vi "LifetimePickTACCube.vi"(2 "notes 2":refnum<vi>, 3 "already x spots":i16) -> (1 "spots":i16)   [LabVIEW 2009]
uses:
  spotproperties.ctl
  <vilib>/vision/NI_Vision_Development_Module.lvlib
panel:
  out "TAC Intensity":u32[](array[numeric])
  out "Lifetime[ns]":ext[](array[numeric]) format="%.2f"
  out "tauerror":dbl[](array[numeric]) format="%.2f"
  out "last coordinates":i32[](array[numeric])
  out "F2-Value overall":dbl format="%.2f"
  out "nachträgliches markieren":i32[](array[numeric]) caption="Coordinates"
  in  "notes":string
  in  "spotsize":bool
  in  "spotsize (Pixel)":u16=10
  out "Intensity":u32[](array[numeric])
  in  "always store button":bool
  out "ALWAYS STORE?":bool
  in  "store this":bool
  out "always store":bool
  in  "Autoscale y":bool caption="Autoscale 2"
  in  "Autoscale":bool
  in  "plot":u16(ring) items=["linear y-axis", "log y-axis"]
  out "takeall?":bool
  out "F2-Value TAC":dbl caption="F2-Value" format="%.2f"
  in  "RGB/false color?":bool
  out "Decays":u32[][](graph)
  out "Tool":i32(ring) items=["Point", "Line", "Rectangle", "Oval", "Polygon", "Free", "Annulus", "Rotated Rectangle", "Zoom", "Pan", "MultiLine", "FreeLine"]
  out "Coordinates":i32[](array[numeric])
  out "Event":i32(ring) items=["No  event", "Click event", "Draw event", "Move event", "Size event", "Scroll event", "Activate event", "Close event", "Double click event"]
  in  "TAC Cube":T1(ring)
  in  "plane":u32
  in  "threshold":cluster{"max":u32, "min":u32} caption="Threshold"
  in  "stop":bool
  # "S"
  # "S"
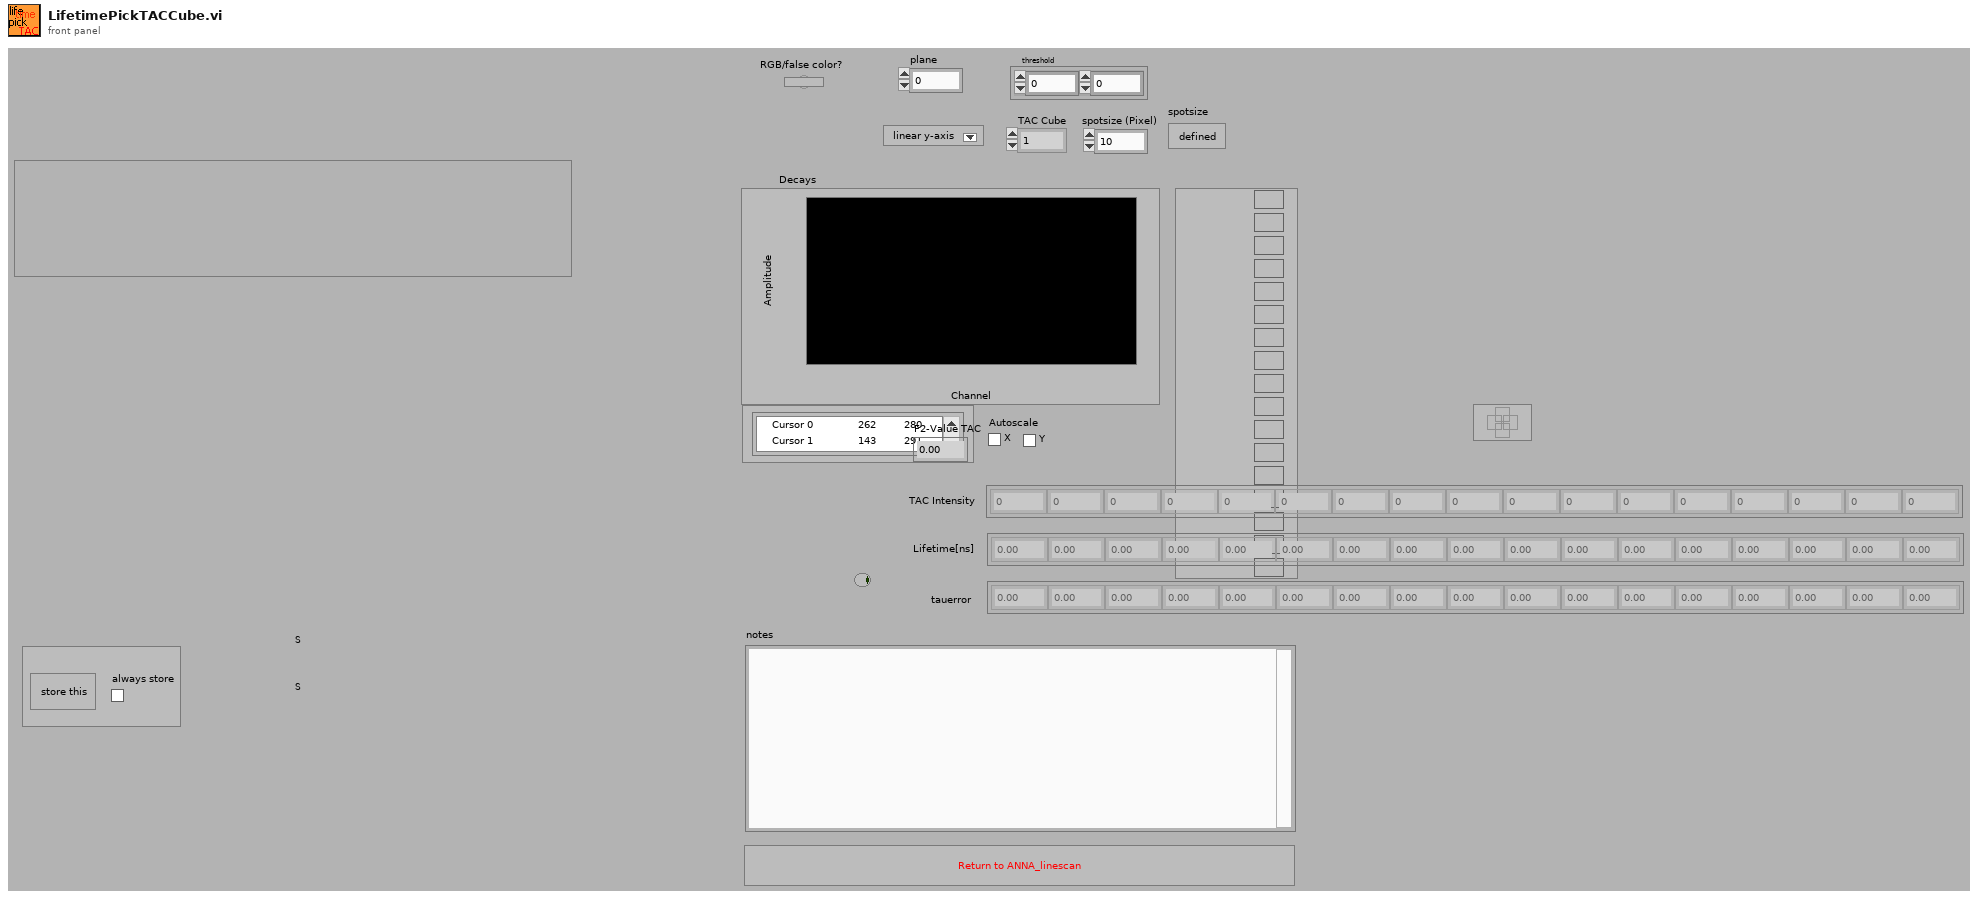
[diagram p1: front panel]
types:
  T1 = enum16{"1", "2", "3", "4", "5", "6", "7", "Sum", "Sep."}
  T2 = typedef "spotproperties.ctl" = cluster{"draw?":bool, "plane":u32, "Coordinates":i32[], "TACWindow":cluster{"TACWindow1":i32, "TACWindow2":i32}, "Lifetime[ns]":ext[], "tauerror":dbl[], "F2-Value overall":dbl, "overall intensity":u32[], "F2-Value TAC":dbl, "TAC intensity":u32[], "Decay":u32[][]}
  T3 = enum16{"Ini", "Get", "Set", "Refresh", "dump", "move", "name"}
  T4 = typedef "FIFOSettings_BH.ctt" = cluster{"Measurement":cluster{"Binning (ms)":sgl, "External Trigger Condition":u16, "Stop Condition:":u16, "Stop Count":dbl, "Buffer Size (Photons)":u16, "No of Channels":u16, "Ext Latch Delay":i16}, "ADC":cluster{"Module":u16, "ADC Resolution":i32, "Dither Range":i16, "Count Increment":i16, "Macro Time Clock":i16}, "SYNC":cluster{"SYNC ZC Level (mV)":sgl, "SYNC Freq Divider":i16, "SYNC Holdoff (ns)":sgl, "SYNC Threshold (mV)":sgl}, "TAC":cluster{"TAC Range (ns)":sgl, "TAC Gain":i16, "TAC Offset (%)":sgl, "TAC Limit Low (%)":sgl, "TAC Limit High (%)":sgl}, "CFD":cluster{"CFD Limit Low (mV)":sgl, "CFD Limit High (mV)":sgl, "CFD ZC Level (mV)":sgl, "CFD Holdoff (ns)":sgl}}
  T5 = typedef "Settings.ctl" = cluster{"threshold":cluster{"max":u32, "min":u32}, "RGB or false color":bool, "16bit":bool, "log/lin axis":u16, "spotsize button":bool, "Pixelsize":u16, "autoscale x":bool, "autoscale y":bool, "correlation":bool, "ADC-Resolution":i32, "F2-lifetime":cluster{"display tau":bool, "display F2":bool, "Palette Number lifetime":enum32{"Gray", "Binary", "Gradient", "Rainbow", "Temperature"}, "Palette Number F2":enum32{"Gray", "Binary", "Gradient", "Rainbow", "Temperature"}, "max tau-Value":dbl, "min tau-Value":dbl, "max F2-Value":dbl, "min F2-Value":dbl}, "TAC-Window 1":u16, "TAC-Window 2":u16, "false color palette":cluster{"1":u32, "2":u32, "3":u32, "4":u32, "5":u32, "6":u32, "7":u32, "8":u32, "8 2":u32, "8 3":u32, "8 4":u32, "8 5":u32}}
  T6 = enum32{"No Selection", "Point", "Line", "Rectangle", "Oval", "Polygon", "Free", "Unused1", "Zoom", "Unused2", "Broken Line", "Free Hand Line"}[]
  T7 = typedef "IMAQ Image.ctl" = refnum<image>
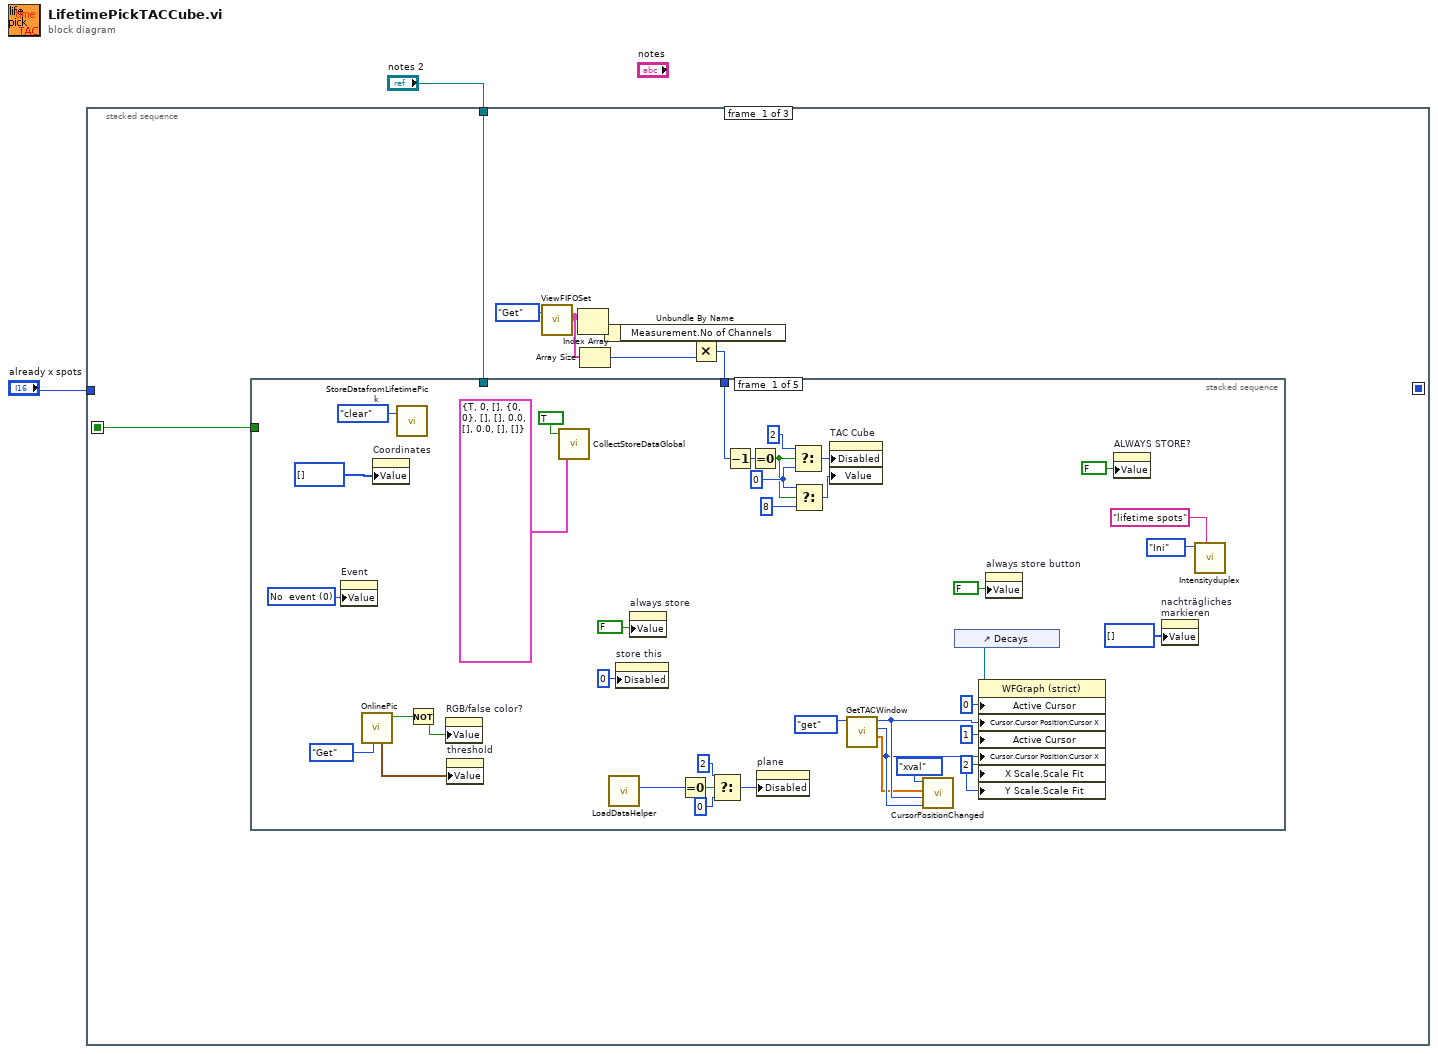
[diagram p0: block diagram]
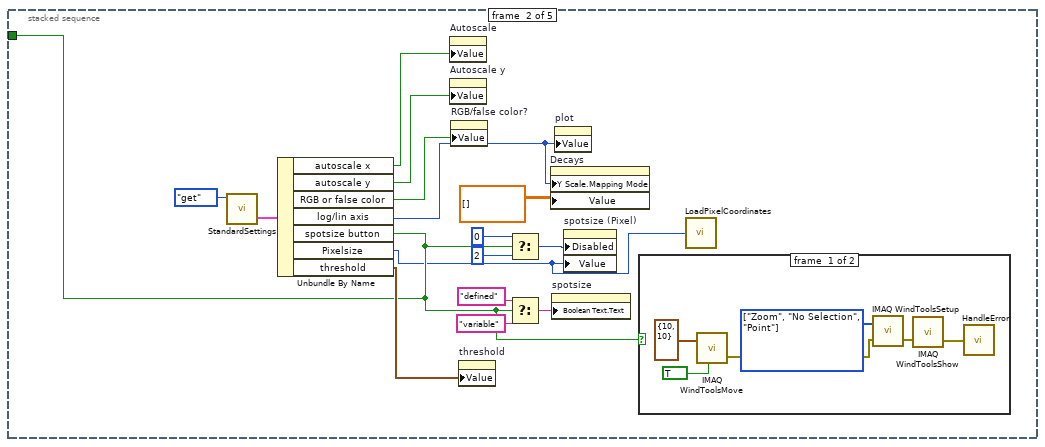
[diagram p2: hidden frame]
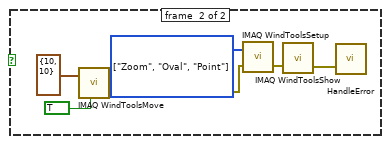
[diagram p3: hidden frame]
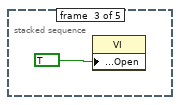
[diagram p4: hidden frame]
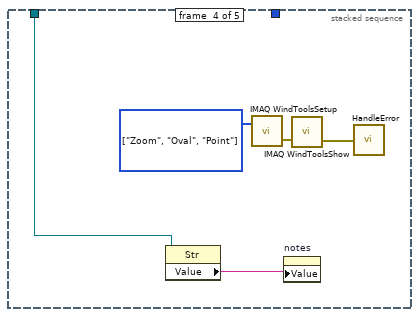
[diagram p5: hidden frame]
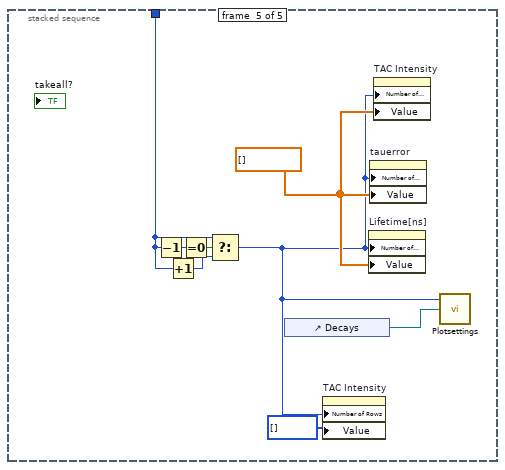
[diagram p6: hidden frame]
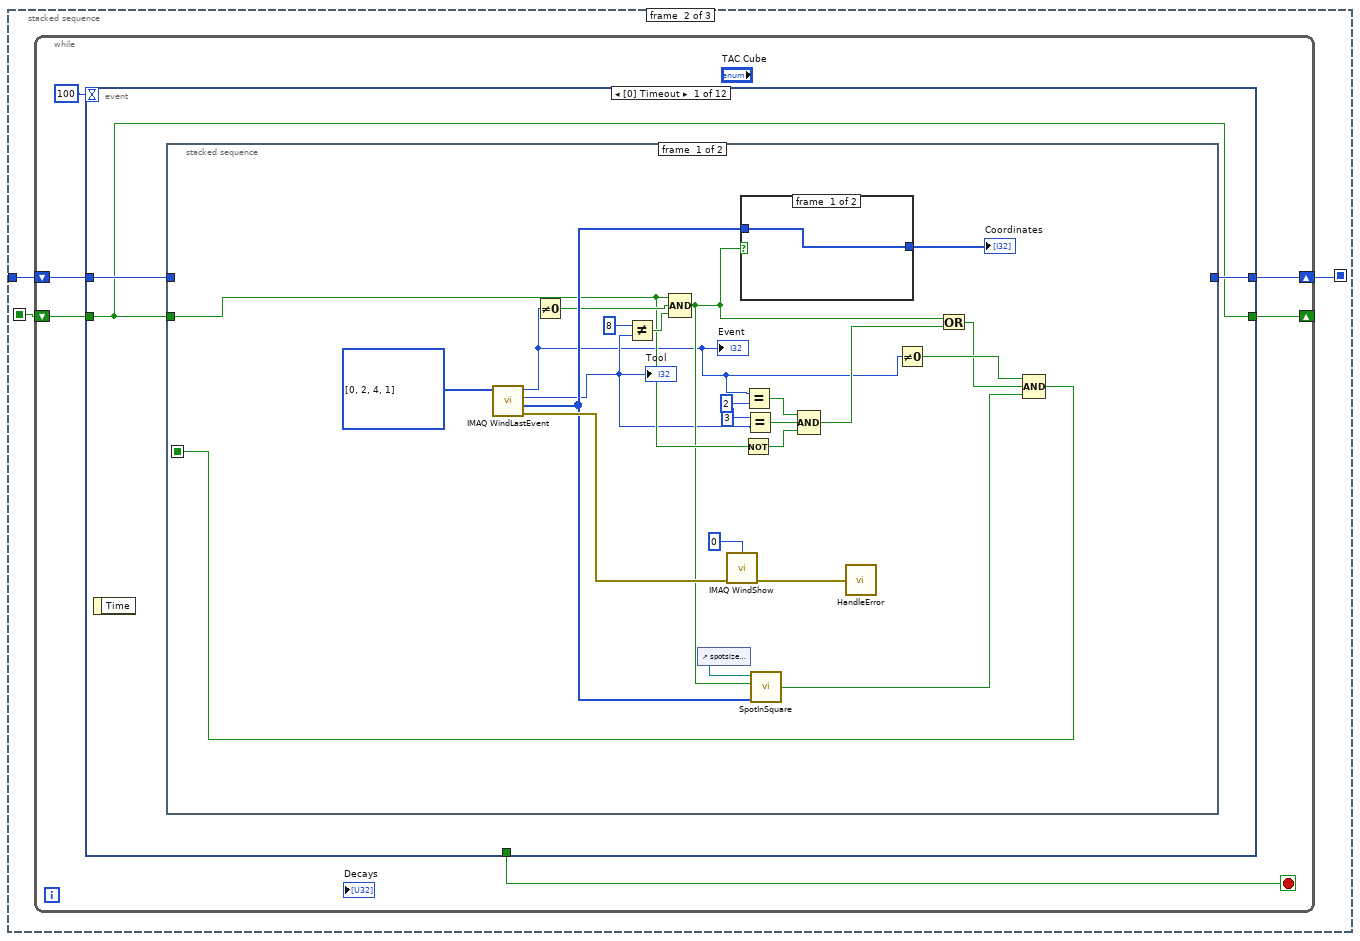
[diagram p7: hidden frame]
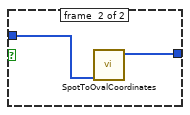
[diagram p8: hidden frame]
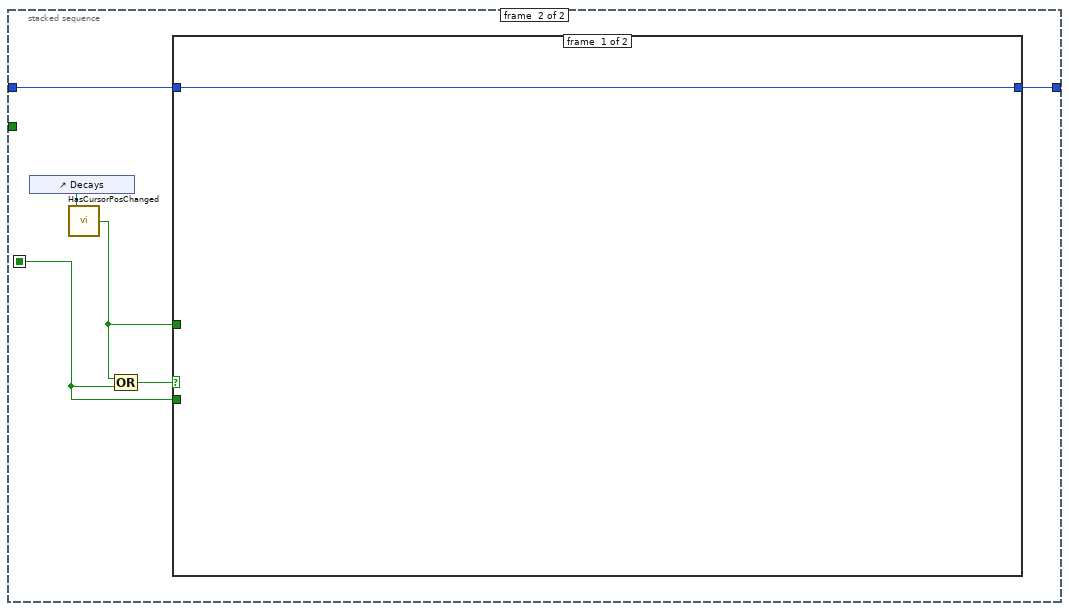
[diagram p9: hidden frame]
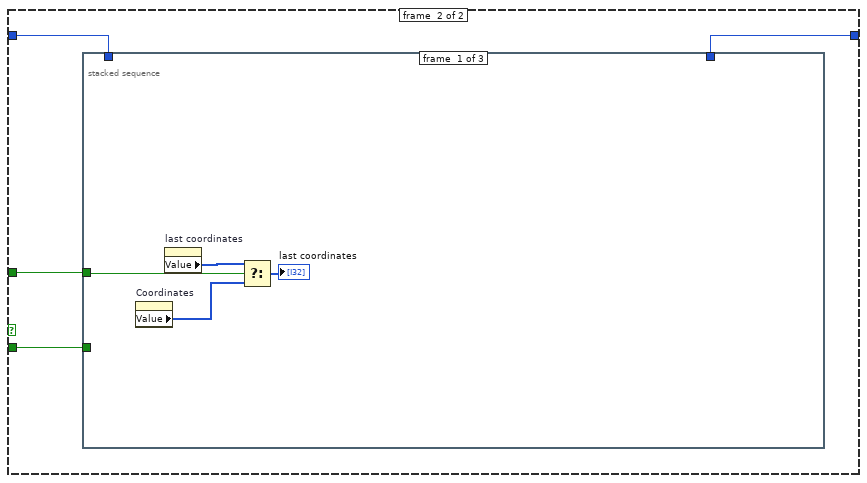
[diagram p10: hidden frame]
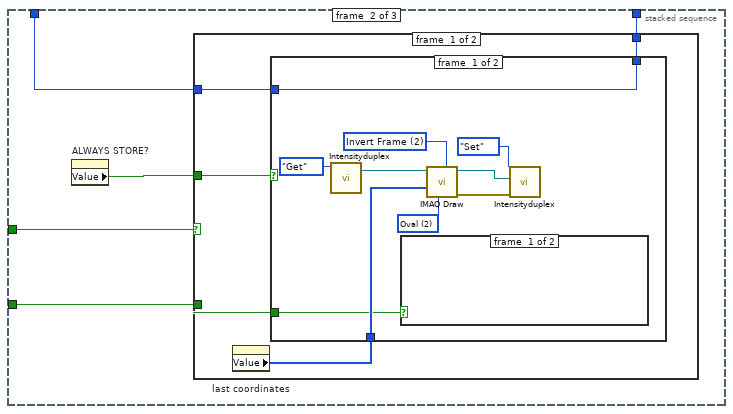
[diagram p11: hidden frame]
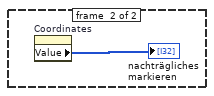
[diagram p12: hidden frame]
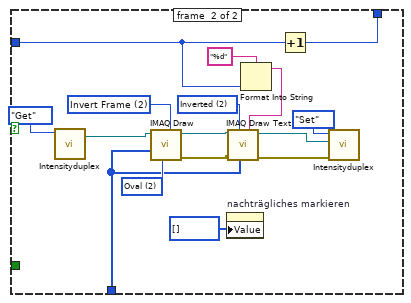
[diagram p13: hidden frame]
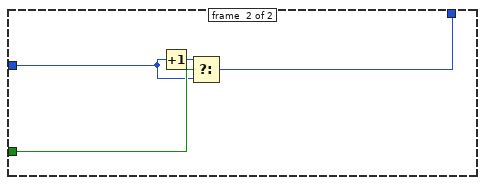
[diagram p14: hidden frame]
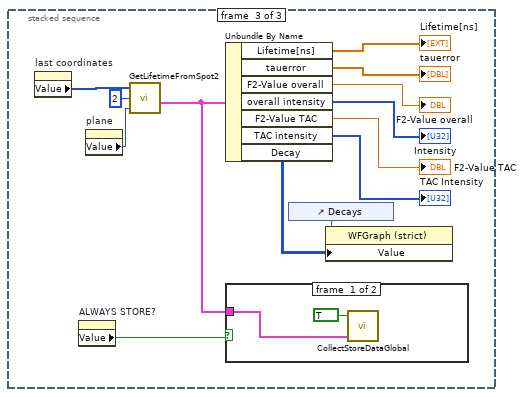
[diagram p15: hidden frame]
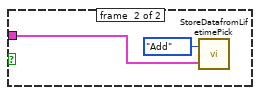
[diagram p16: hidden frame]
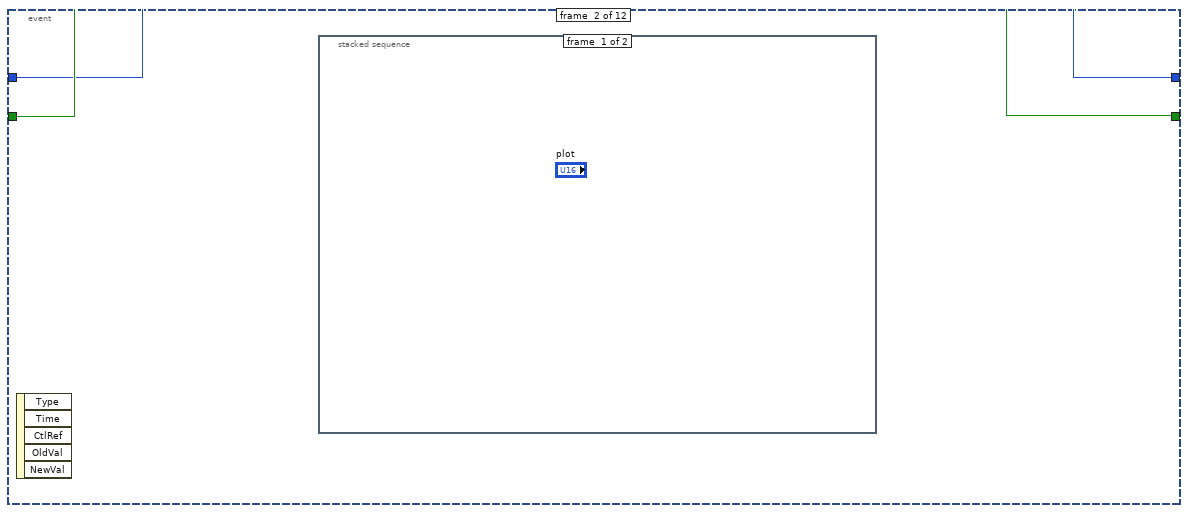
[diagram p17: hidden frame]
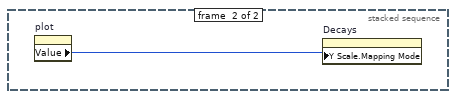
[diagram p18: hidden frame]
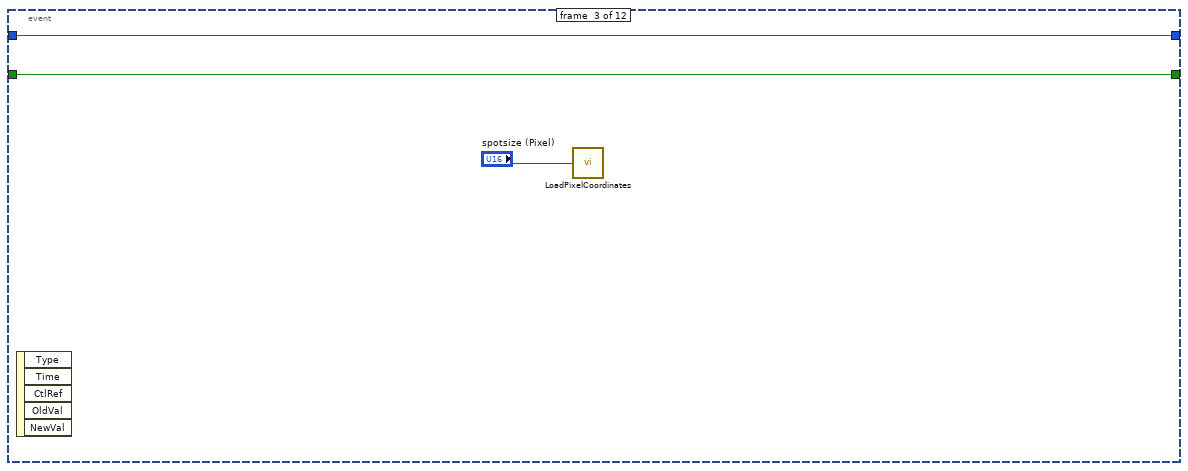
[diagram p19: hidden frame]
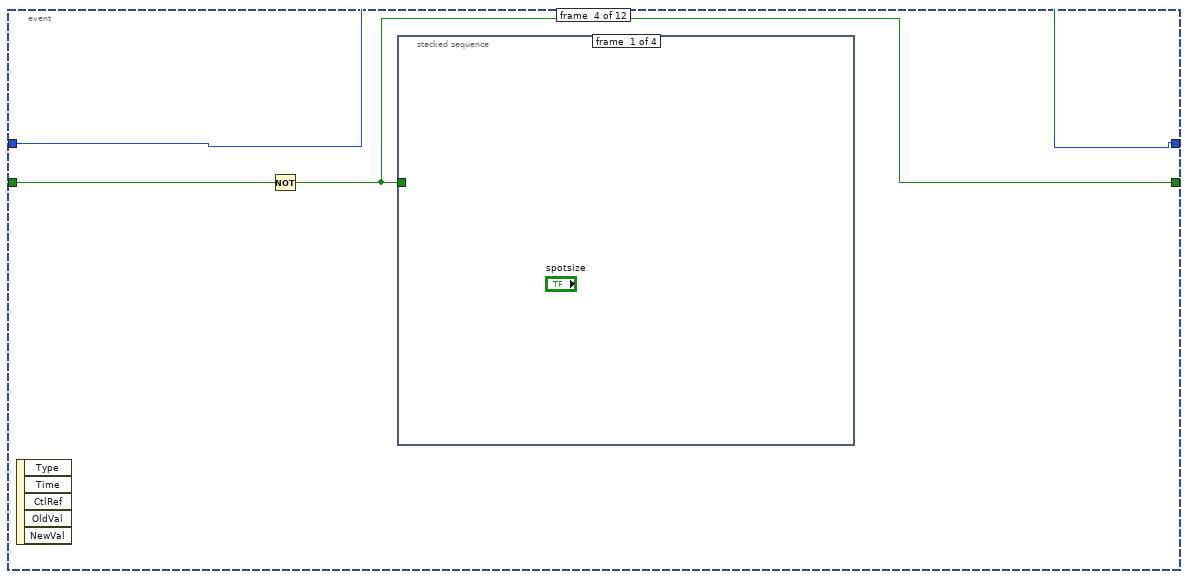
[diagram p20: hidden frame]
diagram:
  n1 = stacked-sequence {
    seq-local: [_ w92 _] -> [_ _ w345]
    seq-local: [w9 _ _] -> [_ w91 _]
    tunnel: "already x spots" -> [_ w93 _]
    tunnel: "notes 2" -> [w10 _ w347]
    frame #0 {
      n2 = call "ViewFIFOSet.vi"("Enum"=enum16{"Display", "change", "Get", "Set"}."Get") -> ("FIFO Settings (Array)"=w6:T4[])  [unwired: 1 in]
      n3 = Index Array(array=w6) -> (element=w7:T4)  [unwired: 1 in]
      n4 = Array Size(array=w6) -> (size(s)=w4:i32)
      n5 = Unbundle By Name(w7) -> ("Measurement.No of Channels"=w3:u16)
      n6 = Multiply(x=w3, y=w4) -> (x*y=w5:i32)
      n7 = stacked-sequence {
        tunnel: w10 -> [_ _ _ w79 _]
        tunnel: [_ w50 _ _ _] -> w9
        tunnel: w5 -> [w13 _ _ _ w86]
        frame #0 {
          w14 = u8 0 ("Disabled")
          w41 = 0 items=["No  event", "Click event", "Draw event", "Move event", "Size event", "Scroll event", "Activate event", "Close event", "Double click event"] ("Event")
          w45 = u8 2 ("X Scale.Scale Fit")
          n8 = property on="Event" class="Ring (strict)"("Value"=w41) -> ()  [unwired: 2 in, 2 out]
          n9 = call "OnlinePic.vi"("action"=enum16{"Get", "Set", "Change", "ini"}."Get" ("Enum")) -> ("RGB/False out"=w32:bool, "Threshold (max) OUT"=w33:cluster{"max":u32, "min":u32})  [unwired: 6 in, 3 out]
          n10 = property on="Coordinates" class="Array (strict)"("Value"=i32[] []) -> ()  [unwired: 2 in, 2 out]
          n11 = call "StoreDatafromLifetimePick.vi"("Enum"=enum16{"clear", "Get", "Set"}."clear") -> ()  [unwired: 1 in, 2 out]
          n12 = Not(x=w32) -> (.not. x?=w31:bool)
          n13 = property on="RGB/false color?" class="Bool (strict)"("Value"=w31) -> ()  [unwired: 2 in, 2 out]
          n14 = property on="threshold" class="Clust (strict)"("Value"=w33) -> ()  [unwired: 2 in, 2 out]
          n15 = call "CollectStoreDataGlobal.vi"("SpotProperties 2"=T2 {"draw?"=TRUE, "plane"=0, "Coordinates"=[], "TACWindow"={"TACWindow1"=0, "TACWindow2"=0}, "Lifetime[ns]"=[], "tauerror"=[], "F2-Value overall"=0.0, "overall intensity"=[], "F2-Value TAC"=0.0, "TAC intensity"=[], "Decay"=[]}, "set?"=TRUE) -> ()  [unwired: 2 in, 1 out]
          n16 = call "LoadDataHelper.vi"() -> ("planes"=w22:u32)  [unwired: 7 in, 4 out]
          n17 = property on="store this" class="Boolean"("Disabled"=u8 0) -> ()  [unwired: 2 in, 2 out]
          n18 = property on="always store" class="Boolean (strict)"("Value"=FALSE ("always store")) -> ()  [unwired: 2 in, 2 out]
          n19 = Equal To 0?(x=w22) -> (x = 0?=w23:bool)
          n20 = Select(t=u8 2 ("Disabled"), s=w23, f=u8 0 ("Disabled")) -> (s? t:f=w19:u8)
          n21 = Decrement(x=w13) -> (x-1=w16:i32)
          n22 = Equal To 0?(x=w16) -> (x = 0?=w12:bool)
          n23 = property on="plane" class="DigNum (strict)"("Disabled"=w19) -> ()  [unwired: 2 in, 2 out]
          n24 = Select(t=u8 2 ("Disabled"), s=w12, f=w14) -> (s? t:f=w17:u8)
          n25 = Select(t=w14, s=w12, f=u8 8) -> (s? t:f=w15:u8)
          n26 = property on="TAC Cube" class="Enum (strict)"("Disabled"=w17, "Value"=w15) -> ()  [unwired: 2 in, 2 out]
          n27 = call "GetTACWindow.vi"("Enum"=enum16{"ini", "get", "quick"}."get") -> ("Cursor.Cursor Position:Cursor X"=w39:u16, "Cursor.Cursor Position:Cursor X 2"=w38:u16, "x-values"=w27:dbl[])  [unwired: 1 in, 6 out]
          n28 = call "CursorPositionChanged.vi"("CursorPos x1"=w38, "CursorPos x0"=w39, "x-values"=w27, "action"=enum16{"Check", "Get", "xval"}."xval" ("Enum")) -> ()  [unwired: 4 out]
          n29 = control-ref of="Decays"() -> (w48:refnum<vi>)
          n30 = property class="WFGraph (strict)"(reference=w48, "Active Cursor"=u32 0, "Cursor.Cursor Position:Cursor X"=w39, "Active Cursor"=u32 1, "Cursor.Cursor Position:Cursor X"=w38, "X Scale.Scale Fit"=w45, "Y Scale.Scale Fit"=w45) -> ()  [unwired: 1 in, 2 out]
          n31 = property on="always store button" class="Bool (strict)"("Value"=FALSE ("always store")) -> ()  [unwired: 2 in, 2 out]
          n32 = property on="ALWAYS STORE?" class="Boolean (strict)"("Value"=FALSE ("ALWAYS STORE?")) -> ()  [unwired: 2 in, 2 out]
          n33 = property on="nachträgliches markieren" class="Arr (strict)"("Value"=i32[] [] ("last Coordinates")) -> ()  [unwired: 2 in, 2 out]
          n34 = call "Intensityduplex.vi"("Enum"=enum16{"Ini", "Get", "Set", "Refresh"}."Ini" ("command"), "title"="lifetime spots") -> ()  [unwired: 3 in, 2 out]
        }
        frame #1 {
          n35 = call "StandardSettings.vi"("Enum"=enum16{"Load", "get", "Save", "set"}."get") -> ("StandardSettings"=w63:T5)  [unwired: 4 in]
          n36 = Unbundle By Name(w63) -> ("autoscale x"=w53:bool, "autoscale y"=w54:bool, "RGB or false color"=w52:bool, "log/lin axis"=w55:u16, "spotsize button"=w50:bool, "Pixelsize"=w49:u16, "threshold"=w51:cluster{"max":u32, "min":u32})
          n37 = property on="Autoscale" class="Boolean (strict)"("Value"=w53) -> ()  [unwired: 2 in, 2 out]
          n38 = property on="Autoscale y" class="Boolean (strict)"("Value"=w54) -> ()  [unwired: 2 in, 2 out]
          n39 = property on="RGB/false color?" class="Boolean (strict)"("Value"=w52) -> ()  [unwired: 2 in, 2 out]
          n40 = property on="threshold" class="Clust (strict)"("Value"=w51) -> ()  [unwired: 2 in, 2 out]
          n41 = Select(t=u8 0, s=w50, f=u8 2) -> (s? t:f=w57:u8)
          n42 = Select(t="defined", s=w50, f="variable") -> (s? t:f=w60:string)
          n43 = property on="Decays" class="WFGraph (strict)"("Y Scale.Mapping Mode"=w55, "Value"=sgl[][] []) -> ()  [unwired: 2 in, 2 out]
          n44 = property on="spotsize" class="Boolean"("Boolean Text.Text"=w60) -> ()  [unwired: 2 in, 2 out]
          n45 = property on="plot" class="Ring (strict)"("Value"=w55) -> ()  [unwired: 2 in, 2 out]
          n46 = property on="spotsize (Pixel)" class="DigNum (strict)"("Disabled"=w57, "Value"=w49) -> ()  [unwired: 2 in, 2 out]
          n47 = case shown="True" w50 {
            frame #0 {
              w70 = T6 [enum."Zoom", enum."No Selection", enum."Point"] items=["No Selection", "Point", "Line", "Rectangle", "Oval", "Polygon", "Free", "Unused1", "Zoom", "Unused2", "Broken Line", "Free Hand Line"] ("Tools")
              n48 = call "IMAQ WindToolsMove"("Coordinates"=cluster{"X Position":i32, "Y Position":i32} {"X Position"=10, "Y Position"=10}, "Get/Set Status? (Set)"=TRUE) -> ("error out"=w66:errorcluster)  [unwired: 3 in, 1 out]
              n49 = call "IMAQ WindToolsSetup"("Tools"=w70, "error in (no error)"=w66) -> ("error out"=w69:errorcluster)  [unwired: 4 in]
              n50 = call "IMAQ WindToolsShow"("error in (no error)"=w69) -> ("error out"=w65:errorcluster)  [unwired: 4 in, 1 out]
              n51 = call "HandleError.vi"("error in (no error)"=w65) -> ()
            }
            frame #1 {
              w76 = T6 [enum."Zoom", enum."Oval", enum."Point"] items=["No Selection", "Point", "Line", "Rectangle", "Oval", "Polygon", "Free", "Unused1", "Zoom", "Unused2", "Broken Line", "Free Hand Line"] ("Tools")
              n52 = call "IMAQ WindToolsMove"("Coordinates"=cluster{"X Position":i32, "Y Position":i32} {"X Position"=10, "Y Position"=10}, "Get/Set Status? (Set)"=TRUE) -> ("error out"=w72:errorcluster)  [unwired: 3 in, 1 out]
              n53 = call "IMAQ WindToolsSetup"("Tools"=w76, "error in (no error)"=w72) -> ("error out"=w75:errorcluster)  [unwired: 4 in]
              n54 = call "IMAQ WindToolsShow"("error in (no error)"=w75) -> ("error out"=w71:errorcluster)  [unwired: 4 in, 1 out]
              n55 = call "HandleError.vi"("error in (no error)"=w71) -> ()
            }
          }
          n56 = call "LoadPixelCoordinates.vi"("spotsize (radius pixel)"=w49) -> ()
        }
        frame #2 {
          n57 = property class="VI"("Front Panel Window:Open"=TRUE) -> ()  [unwired: 2 in, 2 out]
        }
        frame #3 {
          w82 = T6 [enum."Zoom", enum."Oval", enum."Point"] items=["No Selection", "Point", "Line", "Rectangle", "Oval", "Polygon", "Free", "Unused1", "Zoom", "Unused2", "Broken Line", "Free Hand Line"] ("Tools")
          n58 = property class="Str"(reference=w79) -> ("Value"=w80:string)  [unwired: 1 in, 2 out]
          n59 = call "IMAQ WindToolsSetup"("Tools"=w82) -> ("error out"=w81:errorcluster)  [unwired: 5 in]
          n60 = property on="notes" class="String"("Value"=w80) -> ()  [unwired: 2 in, 2 out]
          n61 = call "IMAQ WindToolsShow"("error in (no error)"=w81) -> ("error out"=w78:errorcluster)  [unwired: 4 in, 1 out]
          n62 = call "HandleError.vi"("error in (no error)"=w78) -> ()
        }
        frame #4 {
          w84 = dbl[] []
          n63 = Decrement(x=w86) -> (x-1=w88:i32)
          n64 = Increment(x=w86) -> (x+1=w85:i32)
          n65 = Equal To 0?(x=w88) -> (x = 0?=w87:bool)
          n66 = Select(t=w86, s=w87, f=w85) -> (s? t:f=w83:i32)
          n67 = control-ref of="Decays"() -> (w89:refnum<vi>)
          n68 = property on="TAC Intensity" class="Array (strict)"("Number of Rows"=w83, "Value"=u32[] [] ("TAC Intensity")) -> ()  [unwired: 2 in, 2 out]
          n69 = property on="Lifetime[ns]" class="Array (strict)"("Number of Columns"=w83, "Value"=w84) -> ()  [unwired: 2 in, 2 out]
          n70 = property on="tauerror" class="Array (strict)"("Number of Columns"=w83, "Value"=w84) -> ()  [unwired: 2 in, 2 out]
          n71 = property on="TAC Intensity" class="Array (strict)"("Number of Columns"=w83, "Value"=w84) -> ()  [unwired: 2 in, 2 out]
          n72 = call "Plotsettings.vi"("Decays 2"=w89, "No of Channels"=w83) -> ()  [unwired: 4 in]
        }
      }
    }
    frame #1 {
      n73 = while {
        shift-right: [w96] -> w92
        shift-left: w93 -> [w97]
        shift-right: [w94] -> _
        shift-left: w91 -> [w95]
        stop <- w99 stop-if-true
        n74 = event shown="[0] Timeout" {
          selector: _ -> [_ _ _ _ _ _ _ _ _ _ _ _]
          dyn-events: _ -> [_ _ _ _ _ _ _ _ _ _ _ _]
          timeout: 100 -> [_ _ _ _ _ _ _ _ _ _ _ _]
          tunnel: [_ _ _ _ _ _ _ _ _ _ w326 TRUE] -> w99
          tunnel: w97 -> [w102 w203 w207 w209 w233 w239 w246 w258 w268 w303 w324 w329]
          tunnel: [w101 w203 w207 w209 w233 w239 w246 w258 w267 w302 w324 w329] -> w96
          tunnel: w95 -> [w100 w204 w208 w211 w234 w240 w247 w259 w266 w301 w325 w330]
          tunnel: [w100 w204 w208 w210 w234 w240 w247 w259 w266 w301 w325 w330] -> w94
          event #0 {
            n75 = event-data() -> ()  [unwired: 1 in, 1 out]
            n76 = stacked-sequence {
              seq-local: [w117 _] -> [_ w130]
              tunnel: w102 -> [_ w134]
              tunnel: [_ w133] -> w101
              tunnel: w100 -> [w114 _]
              frame #0 {
                w126 = i32[] [0, 2, 4, 1] items=["No  event", "Click event", "Draw event", "Move event", "Size event", "Scroll event", "Activate event", "Close event", "Double click event"] ("Events list (all)")
                n77 = call "IMAQ WindLastEvent"("Events list (all)"=w126) -> ("error out"=w124:errorcluster, "Coordinates"=w122:i32[], "Tool"=w108:i32, "Event"=w107:i32)  [unwired: 5 in, 2 out]
                "Tool" <- w108
                "Event" <- w107
                n78 = Not Equal To 0?(x=w107) -> (x != 0?=w121:bool)
                n79 = Not Equal?(x=8, y=w108) -> (x != y?=w116:bool)
                n80 = Compound Arithmetic op=AND(w114, w121, w116) -> (w111:bool)
                n81 = control-ref of="spotsize (Pixel)"() -> (w123:refnum<vi>)
                n82 = call "IMAQ WindShow"("error in (no error)"=w124, "Window Number (0...15)"=0) -> ("error out"=w103:errorcluster)  [unwired: 4 in, 2 out]
                n83 = case shown="False" w111 {
                  tunnel: w122 -> [w127 w129]
                  tunnel: [w127 w128] -> w104
                  frame #0 {
                  }
                  frame #1 {
                    n84 = call "SpotToOvalCoordinates.vi"("Spot"=w129) -> ("oval coordinates"=w128:i32[])  [unwired: 4 in, 2 out]
                  }
                }
                "Coordinates" <- w104
                n85 = Not(x=w114) -> (.not. x?=w113:bool)
                n86 = Equal?(x=w107, y=2) -> (x = y?=w109:bool)
                n87 = Equal?(x=3, y=w108) -> (x = y?=w110:bool)
                n88 = call "SpotInSquare.vi"("Coordinates"=w122, "event"=w111, "reference"=w123) -> ("Boolean"=w118:bool)  [unwired: 1 in]
                n89 = Compound Arithmetic op=AND(w109, w110, w113) -> (w112:bool)
                n90 = call "HandleError.vi"("error in (no error)"=w103) -> ()
                n91 = Not Equal To 0?(x=w107) -> (x != 0?=w119:bool)
                n92 = Or(x=w111, y=w112) -> (x .or. y?=w115:bool)
                n93 = Compound Arithmetic op=AND(w119, w115, w118) -> (w117:bool)
              }
              frame #1 {
                n94 = control-ref of="Decays"() -> (w135:refnum<vi>)
                n95 = call "HasCursorPosChanged.vi"("Decay reference"=w135) -> ("changed?"=w132:bool)
                n96 = Compound Arithmetic op=OR(w132, w130) -> (w131:bool)
                n97 = case shown="True" w131 {
                  tunnel: w132 -> [_ w140]
                  tunnel: w134 -> [w136 w139]
                  tunnel: [w136 w138] -> w133
                  tunnel: w130 -> [_ w137]
                  frame #0 {
                  }
                  frame #1 {
                    n98 = stacked-sequence {
                      tunnel: w140 -> [w142 w146 _]
                      tunnel: w139 -> [_ w148 _]
                      tunnel: [_ w149 _] -> w138
                      tunnel: w137 -> [_ w147 _]
                      frame #0 {
                        n99 = property on="Coordinates" class="Arr (strict)"() -> ("Value"=w141:i32[])  [unwired: 2 in, 2 out]
                        n100 = property on="last coordinates" class="Array (strict)"() -> ("Value"=w143:i32[])  [unwired: 2 in, 2 out]
                        n101 = Select(t=w143, s=w142, f=w141) -> (s? t:f=→"last coordinates":i32[])
                      }
                      frame #1 {
                        n102 = property on="ALWAYS STORE?" class="Bool (strict)"() -> ("Value"=w145:bool)  [unwired: 2 in, 2 out]
                        n103 = case shown="False" w146 {
                          tunnel: [w154 w183] -> w149
                          tunnel: w148 -> [w153 w184]
                          tunnel: w147 -> [w152 _]
                          tunnel: w145 -> [w150 w185]
                          frame #0 {
                            n104 = property on="last coordinates" class="Array (strict)"() -> ("Value"=w151:i32[])  [unwired: 2 in, 2 out]
                            n105 = case shown="False" w150 {
                              tunnel: [w164 w181] -> w154
                              tunnel: w153 -> [w164 w173]
                              tunnel: w151 -> [w158 w170]
                              tunnel: w152 -> [w155 _]
                              frame #0 {
                                w162 = u16 2 items=["Frame", "Paint", "Invert Frame", "Invert Paint"] ("Draw Mode")
                                w163 = u16 2 items=["Line", "Rectangle", "Oval"] ("Shape to draw")
                                n106 = call "Intensityduplex.vi"("Enum"=T3."Get") -> ("Image Duplicate (out)"=w161:T7)  [unwired: 4 in, 1 out]
                                n107 = case shown="True" w155 {
                                frame #0 {
                                }
                                frame #1 {
                                n108 = property on="Coordinates" class="Arr (strict)"() -> ("Value"=→"nachträgliches markieren":i32[])  [unwired: 2 in, 2 out]
                                }
                                }
                                n109 = call "IMAQ Draw"("Draw Mode"=w162, "Shape to draw"=w163, "Coordinates"=w158, "Image Src"=w161) -> ("error out"=w159:errorcluster, "Image Dst Out"=w160:T7)  [unwired: 6 in]
                                n110 = call "Intensityduplex.vi"("Enum"=T3."Set", "Image In"=w160, "error in"=w159) -> ()  [unwired: 2 in, 2 out]
                              }
                              frame #1 {
                                w171 = u16 2 items=["Line", "Rectangle", "Oval"] ("Shape to draw")
                                w174 = 2 items=["White", "Black", "Inverted", "Black on White", "White on Black"] ("Color")
                                w175 = u16 2 items=["Frame", "Paint", "Invert Frame", "Invert Paint"] ("Draw Mode")
                                n111 = call "Intensityduplex.vi"("Enum"=T3."Get") -> ("Image Duplicate (out)"=w180:T7)  [unwired: 4 in, 1 out]
                                n112 = call "IMAQ Draw"("Draw Mode"=w175, "Shape to draw"=w171, "Coordinates"=w170, "Image Src"=w180) -> ("error out"=w177:errorcluster, "Image Dst Out"=w179:T7)  [unwired: 6 in]
                                n113 = property on="nachträgliches markieren" class="Arr (strict)"("Value"=i32[] [] ("last Coordinates")) -> ()  [unwired: 2 in, 2 out]
                                n114 = Format Into String(format string="%d", w173) -> (resulting string=w172:string)  [unwired: 2 in, 1 out]
                                n115 = call "IMAQ Draw Text"("String"=w172, "Insertion Point"=w170, "Color"=w174, "error in (no error)"=w177, "Image Src"=w179) -> ("error out"=w176:errorcluster, "Image Dst Out"=w178:T7)  [unwired: 3 in, 2 out]
                                n116 = Increment(x=w173) -> (x+1=w181:i16)
                                n117 = call "Intensityduplex.vi"("Enum"=T3."Set", "Image In"=w178, "error in"=w176) -> ()  [unwired: 2 in, 2 out]
                              }
                            }
                          }
                          frame #1 {
                            n118 = Increment(x=w184) -> (x+1=w182:i16)
                            n119 = Select(t=w182, s=w185, f=w184) -> (s? t:f=w183:i16)
                          }
                        }
                      }
                      frame #2 {
                        n120 = property on="last coordinates" class="Arr (strict)"() -> ("Value"=w186:i32[])  [unwired: 2 in, 2 out]
                        n121 = property on="ALWAYS STORE?" class="Bool (strict)"() -> ("Value"=w190:bool)  [unwired: 2 in, 2 out]
                        n122 = property on="plane" class="DigNum (strict)"() -> ("Value"=w188:u32)  [unwired: 2 in, 2 out]
                        n123 = call "GetLifetimeFromSpot2.vi"("plane"=w188, "F2-channel"=u8 2, "Coordinates"=w186) -> ("SpotProperties"=w189:T2)  [unwired: 5 in]
                        n124 = Unbundle By Name(w189) -> ("Lifetime[ns]"=→"Lifetime[ns]":ext[], "tauerror"=→"tauerror":dbl[], "F2-Value overall"=→"F2-Value overall":dbl, "overall intensity"=→"Intensity":u32[], "F2-Value TAC"=→"F2-Value TAC":dbl, "TAC intensity"=→"TAC Intensity":u32[], "Decay"=w191:u32[][])
                        n125 = case shown="False" w190 {
                          tunnel: w189 -> [w199 w201]
                          frame #0 {
                            (unwired) FALSE
                            n126 = call "CollectStoreDataGlobal.vi"("SpotProperties 2"=w199, "set?"=TRUE) -> ()  [unwired: 2 in, 1 out]
                          }
                          frame #1 {
                            n127 = call "StoreDatafromLifetimePick.vi"("Store Data (input) 2"=w201, "Enum"=enum16{"clear", "Get", "Set", "Add"}."Add") -> ()  [unwired: 2 out]
                          }
                        }
                        n128 = control-ref of="Decays"() -> (w192:refnum<vi>)
                        n129 = property class="WFGraph (strict)"(reference=w192, "Value"=w191) -> ()  [unwired: 1 in, 2 out]
                      }
                    }
                  }
                }
              }
            }
          }
          event #1 {
            n130 = event-data() -> ()  [unwired: 1 in, 5 out]
            n131 = stacked-sequence {
              frame #0 {
              }
              frame #1 {
                n132 = property on="plot" class="Ring (strict)"() -> ("Value"=w205:u16)  [unwired: 2 in, 2 out]
                n133 = property on="Decays" class="WFGraph (strict)"("Y Scale.Mapping Mode"=w205) -> ()  [unwired: 2 in, 2 out]
              }
            }
          }
          event #2 {
            n134 = event-data() -> ()  [unwired: 1 in, 5 out]
            n135 = call "LoadPixelCoordinates.vi"("spotsize (radius pixel)"="spotsize (Pixel)") -> ()
          }
          event #3 {
            n136 = event-data() -> ()  [unwired: 1 in, 5 out]
            n137 = Not(x=w211) -> (.not. x?=w210:bool)
            n138 = stacked-sequence {
              tunnel: w210 -> [_ w212 w219 w220]
              frame #0 {
              }
              frame #1 {
                n139 = Select(t="defined", s=w212, f="variable") -> (s? t:f=w213:string)
                n140 = property on="spotsize" class="Boolean"("Boolean Text.Text"=w213) -> ()  [unwired: 2 in, 2 out]
              }
              frame #2 {
                n141 = Select(t=0, s=w219, f=2) -> (s? t:f=w216:i32)
                n142 = property on="spotsize (Pixel)" class="DigNum (strict)"("Disabled"=w216) -> ()  [unwired: 2 in, 2 out]
              }
              frame #3 {
                n143 = case shown="False" w220 {
                  frame #0 {
                    w226 = T6 [enum."Zoom", enum."No Selection", enum."Point"] items=["No Selection", "Point", "Line", "Rectangle", "Oval", "Polygon", "Free", "Unused1", "Zoom", "Unused2", "Broken Line", "Free Hand Line"] ("Tools")
                    n144 = call "IMAQ WindToolsMove"("Coordinates"=cluster{"X Position":i32, "Y Position":i32} {"X Position"=10, "Y Position"=10}, "Get/Set Status? (Set)"=TRUE) -> ("error out"=w222:errorcluster)  [unwired: 3 in, 1 out]
                    n145 = call "IMAQ WindToolsSetup"("Tools"=w226, "error in (no error)"=w222) -> ("error out"=w225:errorcluster)  [unwired: 4 in]
                    n146 = call "IMAQ WindToolsShow"("error in (no error)"=w225) -> ("error out"=w221:errorcluster)  [unwired: 4 in, 1 out]
                    n147 = call "HandleError.vi"("error in (no error)"=w221) -> ()
                  }
                  frame #1 {
                    w232 = T6 [enum."Zoom", enum."Oval", enum."Point"] items=["No Selection", "Point", "Line", "Rectangle", "Oval", "Polygon", "Free", "Unused1", "Zoom", "Unused2", "Broken Line", "Free Hand Line"] ("Tools")
                    n148 = call "IMAQ WindToolsMove"("Coordinates"=cluster{"X Position":i32, "Y Position":i32} {"X Position"=10, "Y Position"=10}, "Get/Set Status? (Set)"=TRUE) -> ("error out"=w228:errorcluster)  [unwired: 3 in, 1 out]
                    n149 = call "IMAQ WindToolsSetup"("Tools"=w232, "error in (no error)"=w228) -> ("error out"=w231:errorcluster)  [unwired: 4 in]
                    n150 = call "IMAQ WindToolsShow"("error in (no error)"=w231) -> ("error out"=w227:errorcluster)  [unwired: 4 in, 1 out]
                    n151 = call "HandleError.vi"("error in (no error)"=w227) -> ()
                  }
                }
              }
            }
          }
          event #4 {
            n152 = event-data() -> ()  [unwired: 1 in, 5 out]
            n153 = case shown="True" "Autoscale" {
              tunnel: [0 2] -> w236
              frame #0 {
              }
              frame #1 {
              }
            }
            n154 = property on="Autoscale" class="Boolean (strict)"("Value"="Autoscale") -> ()  [unwired: 2 in, 2 out]
            n155 = property on="Decays" class="WFGraph (strict)"("X Scale.Scale Fit"=w236) -> ()  [unwired: 2 in, 2 out]
          }
          event #5 {
            n156 = event-data() -> ()  [unwired: 1 in, 5 out]
            n157 = case shown="True" "Autoscale y" {
              tunnel: [0 2] -> w242
              frame #0 {
              }
              frame #1 {
              }
            }
            n158 = property on="Autoscale y" class="Boolean (strict)"("Value"="Autoscale y") -> ()  [unwired: 2 in, 2 out]
            n159 = property on="Decays" class="WFGraph (strict)"("Y Scale.Scale Fit"=w242) -> ()  [unwired: 2 in, 2 out]
          }
          event #6 {
            n160 = event-data() -> ()  [unwired: 1 in, 5 out]
            n161 = property on="plane" class="DigNum (strict)"() -> ("Value"=w249:u32)  [unwired: 2 in, 2 out]
            n162 = property on="threshold" class="Clust (strict)"() -> ("Value"=w248:cluster{"max":u32, "min":u32})  [unwired: 2 in, 2 out]
            n163 = call "OnlinePic.vi"("action"=enum16{"Get", "Set", "Change", "ini"}."Change" ("Enum"), "RGB/False"="RGB/false color?", "Threshold (max)"=w248, "plane"=w249, "router channel"=u16 0) -> ()  [unwired: 2 in, 5 out]
          }
          event #7 {
            n164 = event-data() -> ()  [unwired: 1 in, 5 out]
            n165 = Unbundle By Name("threshold") -> ("max"=w257:u32, "min"=w256:u32)
            n166 = Max & Min(x=w257, y=w256) -> (max(x,y)=w255:u32, min(x,y)=w254:u32)
            n167 = property on="RGB/false color?" class="Boolean (strict)"() -> ("Value"=w261:bool)  [unwired: 2 in, 2 out]
            n168 = Bundle By Name(cluster="threshold", "max"=w255, "min"=w254) -> (w252:cluster{"max":u32, "min":u32})
            n169 = call "OnlinePic.vi"("action"=enum16{"Get", "Set", "Change", "ini"}."Change" ("Enum"), "RGB/False"=w261, "Threshold (max)"=w252, "plane"="plane") -> ()  [unwired: 3 in, 5 out]
            n170 = property on="threshold" class="Cluster (strict)"("Value"=w252) -> ()  [unwired: 2 in, 2 out]
          }
          event #8 {
            n171 = event-data() -> ()  [unwired: 1 in, 5 out]
            n172 = property on="nachträgliches markieren" class="Array (strict)"() -> ("Value"=w263:i32[])  [unwired: 2 in, 2 out]
            n173 = Add Array Elements(numeric array=w263) -> (sum=w265:i32)
            n174 = Not Equal To 0?(x=w265) -> (x != 0?=w264:bool)
            n175 = stacked-sequence {
              tunnel: w268 -> [_ _ w278 _ _]
              tunnel: [_ _ w277 _ _] -> w267
              tunnel: w264 -> [_ _ w276 w291 _]
              tunnel: w263 -> [_ _ w275 _ _]
              frame #0 {
                n176 = property on="ALWAYS STORE?" class="Boolean (strict)"() -> ("Value"=w270:bool)  [unwired: 2 in, 2 out]
                n177 = Not(x=w270) -> (.not. x?=→"always store" →"ALWAYS STORE?":bool)
              }
              frame #1 {
                n178 = property on="ALWAYS STORE?" class="Boolean (strict)"() -> ("Value"=w274:bool)  [unwired: 2 in, 2 out]
                n179 = Select(t=u8 2 ("Disabled"), s=w274, f=u8 0 ("Disabled")) -> (s? t:f=w273:u8)
                n180 = property on="store this" class="Boolean"("Disabled"=w273) -> ()  [unwired: 2 in, 2 out]
              }
              frame #2 {
                n181 = case shown="True" w276 {
                  tunnel: w278 -> [w279 w285]
                  tunnel: [w279 w284] -> w277
                  tunnel: w275 -> [_ w282]
                  frame #0 {
                  }
                  frame #1 {
                    w289 = 2 items=["White", "Black", "Inverted", "Black on White", "White on Black"] ("Color")
                    n182 = call "Intensityduplex.vi"("Enum"=T3."Get") -> ("Image Duplicate (out)"=w286:T7)  [unwired: 4 in, 1 out]
                    n183 = Format Into String(format string="%d", w285) -> (resulting string=w290:string)  [unwired: 2 in, 1 out]
                    n184 = call "IMAQ Draw Text"("String"=w290, "Insertion Point"=w282, "Color"=w289, "Image Src"=w286) -> ("error out"=w288:errorcluster, "Image Dst Out"=w287:T7)  [unwired: 4 in, 2 out]
                    n185 = call "Intensityduplex.vi"("Enum"=T3."Set", "Image In"=w287, "error in"=w288) -> ()  [unwired: 2 in, 2 out]
                    n186 = Increment(x=w285) -> (x+1=w284:i16)
                  }
                }
              }
              frame #3 {
                n187 = property on="ALWAYS STORE?" class="Boolean (strict)"() -> ("Value"=w292:bool)  [unwired: 2 in, 2 out]
                n188 = And(x=w292, y=w291) -> (x .and. y?=w293:bool)
                n189 = case shown="True" w293 {
                  frame #0 {
                  }
                  frame #1 {
                    n190 = call "CollectStoreDataGlobal.vi"("set?"=FALSE) -> ("SpotProperties"=w295:T2)  [unwired: 3 in]
                    n191 = call "StoreDatafromLifetimePick.vi"("Store Data (input) 2"=w295, "Enum"=enum16{"clear", "Get", "Set", "Add"}."Add") -> ()  [unwired: 2 out]
                  }
                }
              }
              frame #4 {
                n192 = property on="nachträgliches markieren" class="Array (strict)"("Value"=i32[] [] ("last Coordinates")) -> ()  [unwired: 2 in, 2 out]
              }
            }
          }
          event #9 {
            n193 = event-data() -> ()  [unwired: 1 in, 5 out]
            n194 = property on="nachträgliches markieren" class="Arr (strict)"() -> ("Value"=w298:i32[])  [unwired: 2 in, 2 out]
            n195 = Add Array Elements(numeric array=w298) -> (sum=w300:i32)
            n196 = Not Equal To 0?(x=w300) -> (x != 0?=w299:bool)
            n197 = stacked-sequence {
              tunnel: w303 -> [_ _ w311 _]
              tunnel: [_ _ w310 _] -> w302
              tunnel: w299 -> [_ w304 w309 _]
              tunnel: w298 -> [_ _ w308 _]
              frame #0 {
              }
              frame #1 {
                n198 = case shown="True" w304 {
                  frame #0 {
                  }
                  frame #1 {
                    n199 = call "CollectStoreDataGlobal.vi"("set?"=FALSE) -> ("SpotProperties"=w306:T2)  [unwired: 3 in]
                    n200 = call "StoreDatafromLifetimePick.vi"("Store Data (input) 2"=w306, "Enum"=enum16{"clear", "Get", "Set", "Add"}."Add") -> ()  [unwired: 2 out]
                  }
                }
              }
              frame #2 {
                n201 = case shown="True" w309 {
                  tunnel: w308 -> [_ w322]
                  tunnel: w311 -> [w312 w317]
                  tunnel: [w312 w316] -> w310
                  frame #0 {
                  }
                  frame #1 {
                    w320 = 2 items=["White", "Black", "Inverted", "Black on White", "White on Black"] ("Color")
                    n202 = call "Intensityduplex.vi"("Enum"=T3."Get") -> ("Image Duplicate (out)"=w315:T7)  [unwired: 4 in, 1 out]
                    n203 = Format Into String(w317) -> (resulting string=w321:string)  [unwired: 3 in, 1 out]
                    n204 = call "IMAQ Draw Text"("String"=w321, "Insertion Point"=w322, "Color"=w320, "Image Src"=w315) -> ("error out"=w319:errorcluster, "Image Dst Out"=w318:T7)  [unwired: 4 in, 2 out]
                    n205 = Increment(x=w317) -> (x+1=w316:i16)
                    n206 = call "Intensityduplex.vi"("Enum"=T3."Set", "Image In"=w318, "error in"=w319) -> ()  [unwired: 2 in, 2 out]
                  }
                }
              }
              frame #3 {
                n207 = property on="nachträgliches markieren" class="Array (strict)"("Value"=i32[] [] ("last Coordinates")) -> ()  [unwired: 2 in, 2 out]
              }
            }
          }
          event #10 {
            n208 = event-data() -> ()  [unwired: 1 in, 5 out]
            n209 = stacked-sequence {
              tunnel: [_ _ TRUE] -> w326
              frame #0 {
              }
              frame #1 {
                n210 = property class="VI"("Front Panel Window:Open"=FALSE) -> ()  [unwired: 2 in, 2 out]
              }
              frame #2 {
              }
            }
          }
          event #11 {
            n211 = event-data() -> ()  [unwired: 1 in, 3 out]
            n212 = event-data("Discard?"=FALSE) -> ()  [unwired: 1 in, 1 out]
          }
        }
      }
    }
    frame #2 {
      n213 = property on="spotsize (Pixel)" class="DigNum (strict)"() -> ("Disabled"=w339:u8, "Value"=w335:u16)  [unwired: 2 in, 2 out]
      n214 = property on="threshold" class="Clust (strict)"() -> ("Value"=w340:cluster{"max":u32, "min":u32})  [unwired: 2 in, 2 out]
      n215 = property on="RGB/false color?" class="Boolean (strict)"() -> ("Value"=w338:bool)  [unwired: 2 in, 2 out]
      n216 = property on="plot" class="Ring (strict)"() -> ("Value"=w337:u16)  [unwired: 2 in, 2 out]
      n217 = property on="Autoscale" class="Boolean (strict)"() -> ("Value"=w334:bool)  [unwired: 2 in, 2 out]
      n218 = property on="Autoscale y" class="Boolean (strict)"() -> ("Value"=w333:bool)  [unwired: 2 in, 2 out]
      n219 = property on="notes" class="String"() -> ("Value"=w346:string)  [unwired: 2 in, 2 out]
      n220 = Equal To 0?(x=w339) -> (x = 0?=w336:bool)
      n221 = call "StandardSettings.vi"("Enum"=enum16{"Load", "get", "Save", "set"}."get") -> ("StandardSettings"=w341:T5)  [unwired: 4 in]
      n222 = property class="Str"(reference=w347, "Value"=w346) -> ()  [unwired: 1 in, 2 out]
      n223 = Bundle By Name(cluster=w341, "threshold"=w340, "RGB or false color"=w338, "log/lin axis"=w337, "spotsize button"=w336, "Pixelsize"=w335, "autoscale x"=w334, "autoscale y"=w333) -> (w342:T5)
      n224 = call "StandardSettings.vi"("StandardSettings"=w342, "Enum"=enum16{"Load", "get", "Save", "set"}."set") -> ()  [unwired: 3 in, 1 out]
      "spots" <- w345
    }
  }
